vi "LWXPS_PositionerCorrectorPIDFFVelocityGet.vi"(0 "XPS Reference IN":refnum<k24>, 2 "Positioner Name":string, 7 "LabVIEW error IN":errorcluster) -> (12 "XPS Reference OUT":refnum<k24>, 13 "LabVIEW error OUT":errorcluster, 14 "Returned error code":i32, 15 "XPS Error String":string, 16 "Closed Loop Status":bool, 17 "Feed forward velocity":dbl, 18 "Proportional gain":dbl, 19 "Form coefficient":dbl, 20 "Integral gain":dbl, 21 "Derivative gain":dbl, 22 "Integral saturation value":dbl, 23 "Integration time":dbl, 24 "Derivative filter cut off frequency":dbl, 25 "Proportional gain multiplier":dbl, 26 "Integral gain multiplier":dbl, 27 "Derivative gain multiplier":dbl)   [LabVIEW 2014]
uses:
  D:/XPSQ8_LabView_Library/Development/Source/Dll/Newport.XPS.CommandInterface.dll
  Dll/Newport.XPS.CommandInterface.dll
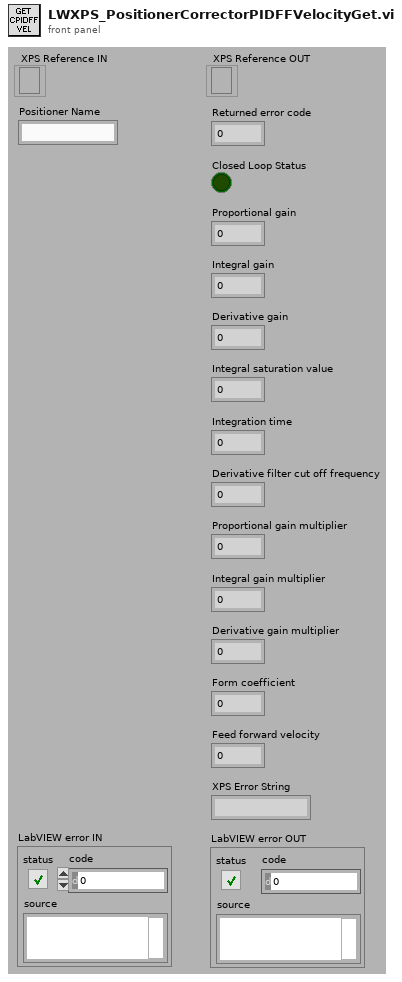
[diagram p1: front panel]
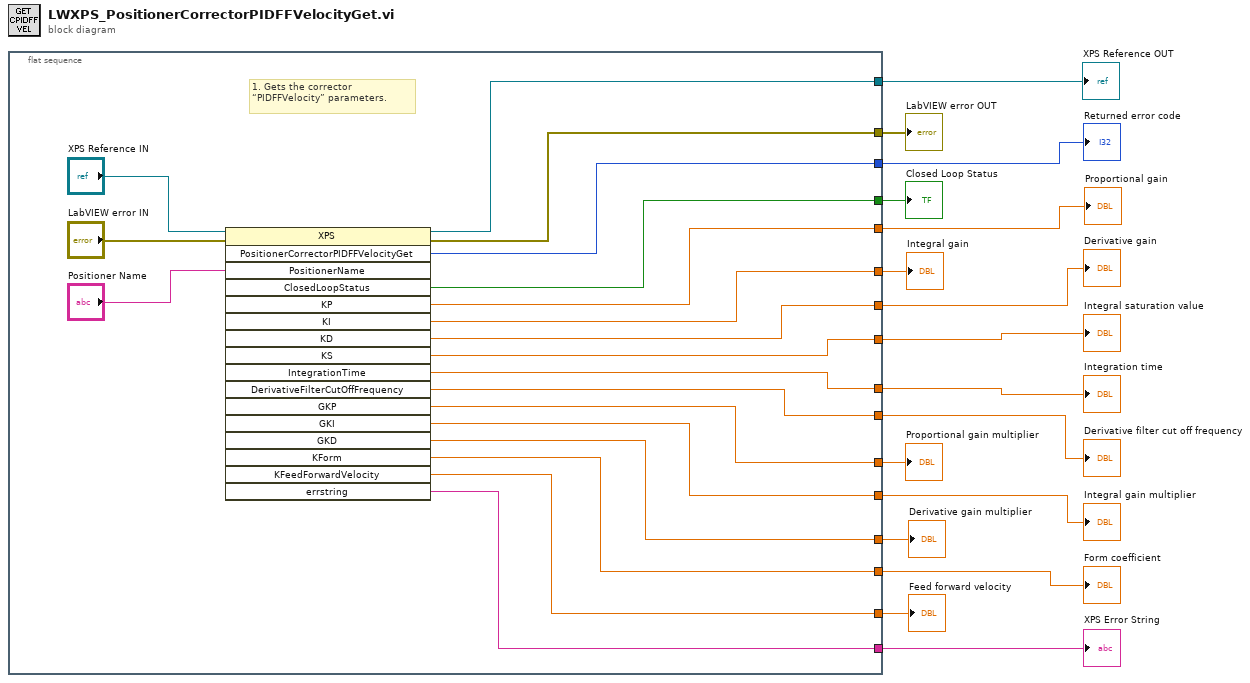
[diagram p0: block diagram]
diagram:
  n1 = flat-sequence {
    tunnel: [w33] -> w7
    tunnel: [w26] -> w16
    tunnel: [w34] -> w15
    tunnel: [w30] -> w14
    tunnel: [w29] -> w13
    tunnel: [w27] -> w12
    tunnel: [w28] -> w11
    tunnel: [w21] -> w10
    tunnel: [w25] -> w8
    tunnel: [w24] -> w2
    tunnel: [w23] -> w9
    tunnel: [w22] -> w3
    tunnel: [w20] -> w6
    tunnel: [w19] -> w5
    tunnel: [w18] -> w4
    tunnel: [w17] -> w1
    frame #0 {
      # "1. Gets the corrector “PIDFFVelocity” parameters."
      n2 = invoke class="XPS" method="PositionerCorrectorPIDFFVelocityGet"(reference="XPS Reference IN", error in="LabVIEW error IN", "PositionerName"="Positioner Name") -> (reference out=w33:refnum<k24>, error out=w26:errorcluster, "PositionerCorrectorPIDFFVelocityGet"=w34:i32, "ClosedLoopStatus"=w25:bool, "KP"=w30:dbl, "KI"=w29:dbl, "KD"=w27:dbl, "KS"=w28:dbl, "IntegrationTime"=w21:dbl, "DerivativeFilterCutOffFrequency"=w24:dbl, "GKP"=w23:dbl, "GKI"=w22:dbl, "GKD"=w20:dbl, "KForm"=w19:dbl, "KFeedForwardVelocity"=w18:dbl, "errstring"=w17:string)  [unwired: 14 in, 1 out]
    }
  }
  "XPS Error String" <- w1
  "XPS Reference OUT" <- w7
  "LabVIEW error OUT" <- w16
  "Returned error code" <- w15
  "Proportional gain" <- w14
  "Integral gain" <- w13
  "Derivative gain" <- w12
  "Integral saturation value" <- w11
  "Integration time" <- w10
  "Derivative filter cut off frequency" <- w2
  "Proportional gain multiplier" <- w9
  "Closed Loop Status" <- w8
  "Derivative gain multiplier" <- w6
  "Form coefficient" <- w5
  "Feed forward velocity" <- w4
  "Integral gain multiplier" <- w3
